vi "Stop Core.vi"(10 "final error code":i32, 11 "Timing Engine Tester in":refnum<class "Timing Engine Tester.lvclass">) -> (3 "Timing Engine Tester out":refnum<class "Timing Engine Tester.lvclass">)   [LabVIEW 2016, in "Timing Engine Tester.lvlib" / "Timing Engine Tester.lvclass"]
doc: "(<B>Filename</B>: Actor Framework.lvlib:Actor.lvclass:Stop Core.vi)\n\nDefines what the actor does before it stops. Use the <B>final error code</B> input to determine whether the actor shut down in response to an error.\n\nBy default, this method does nothing. A descendant class may override it to define behavior, such as shutting down any processes the actor initiated in its override of the Actor Core method."
uses:
  Timing Engine Tester.lvclass
  Timing Engine Tester.lvclass/Timing Engine Tester.ctl
  Core/Base UI Actor/Base UI Actor/Base UI Actor.lvclass
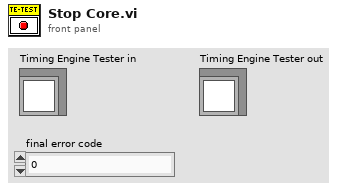
[diagram p1: front panel]
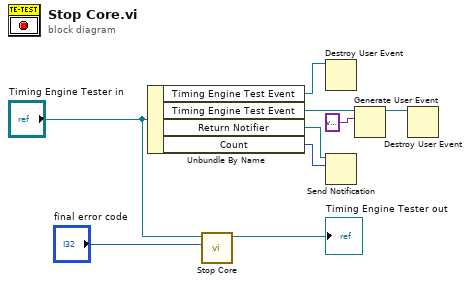
[diagram p0: block diagram]
diagram:
  n1 = Unbundle By Name("Timing Engine Tester in") -> ("Timing Engine Test Event"=w6:refnum<user-event>, "Timing Engine Test Event"=w5:refnum<user-event>, "Return Notifier"=w2:refnum<notifier>, "Count"=w1:i32)
  n2 = call-parent "Stop Core.vi"("final error code"="final error code", "Base UI Actor in"="Timing Engine Tester in") -> ("Base UI Actor out"=→"Timing Engine Tester out":refnum<class "Timing Engine Tester.lvclass">)  [unwired: 9 in]
  n3 = Destroy User Event(user event=w6) -> ()  [unwired: 1 in, 1 out]
  n4 = Send Notification(notification=w1, notifier=w2) -> ()  [unwired: 1 in, 2 out]
  n5 = Generate User Event(user event=w5, event data cluster=variant ("event data")) -> (user event out=w4:refnum<user-event>)  [unwired: 2 in, 1 out]
  n6 = Destroy User Event(user event=w4) -> ()  [unwired: 1 in, 1 out]
